vi "Test_Class.vi"() -> ()   [LabVIEW 2023, in "Picture2D.lvlib"]
uses:
  Picture2D/Picture2D.lvlib
  Circle/Circle.lvclass
  C:/GitHub/Picture2D/src/Shape/Shape.lvclass
  C:/GitHub/Picture2D/src/IDrawable/IDrawable.lvclass
  PointSpecialized/PointSpecialized.lvclass
  C:/GitHub/Picture2D/src/Point/Point.lvclass
  Collection/Collection.lvclass
  ColorHSL/ColorHSL.lvclass
  C:/GitHub/Picture2D/src/Color/Color.lvclass
  Pen/Pen.lvclass
  Picture/Image.lvclass
  Line/Line.lvclass
  Rectangle/Rectangle.lvclass
  C:/GitHub/Picture2D/src/Polygone/Polygone.lvclass
  Text/Text.lvclass
  C:/GitHub/Picture2D/src/Picture2D/Picture2D.lvclass
  Square/Square.lvclass
  RoundRectangle/RoundRectangle.lvclass
  C:/GitHub/Picture2D/src/Rectangle/Rectangle.lvclass
  Point/Point.lvclass
  Color/Color.lvclass
  Triangle/Triangle.lvclass
  Losange/Losange.lvclass
  TriangleR/TriangleR.lvclass
  C:/GitHub/Picture2D/src/Triangle/Triangle.lvclass
  Font/Font.lvclass
  UMLClass/UMLClass.lvclass
  TriangleL/TriangleL.lvclass
  TriangleB/TriangleB.lvclass
  GrayScaleImage/GrayScaleImage.lvclass
  C:/GitHub/Picture2D/src/Picture/Image.lvclass
  2DPictureControl/2DPictureControl.lvclass
  Font/Font.lvclass/Font.ctl
  UMLClass/UMLClass.lvclass/UMLClass.ctl
  PointSpecialized/PointSpecialized.lvclass/PointSpecialized.ctl
  Font/SetFontName.vi
  Font/SetSize.vi
  UMLClass/SetClassName.vi
  UMLClass/SetMethods.vi
  UMLClass/SetProperties.vi
  PointSpecialized/SetColor.vi
  PointSpecialized/SetPen.vi
panel:
  in  "Num Px":i16=1
  in  "Down":bool
  in  "Right":bool
  in  "Left":bool
  in  "Up":bool
  in  "Reinit":bool
  in  "Zoom Factor":dbl(slide)=1.0 scale=0.5..3.0
  in  "Fill":bool
  in  "Rotate (deg)":dbl(slide)=1.0 scale=-180.0..180.0
  in  "Point:y":i16(slide) scale=-100.0..100.0
  in  "Point:x":i16(slide) scale=-100.0..100.0
  in  "Scale Factor":dbl(slide)=1.0 scale=0.5..2.0
  out "2D Picture out":picture
  # "Move Absolute"
  # "Move Relative (1 px)"
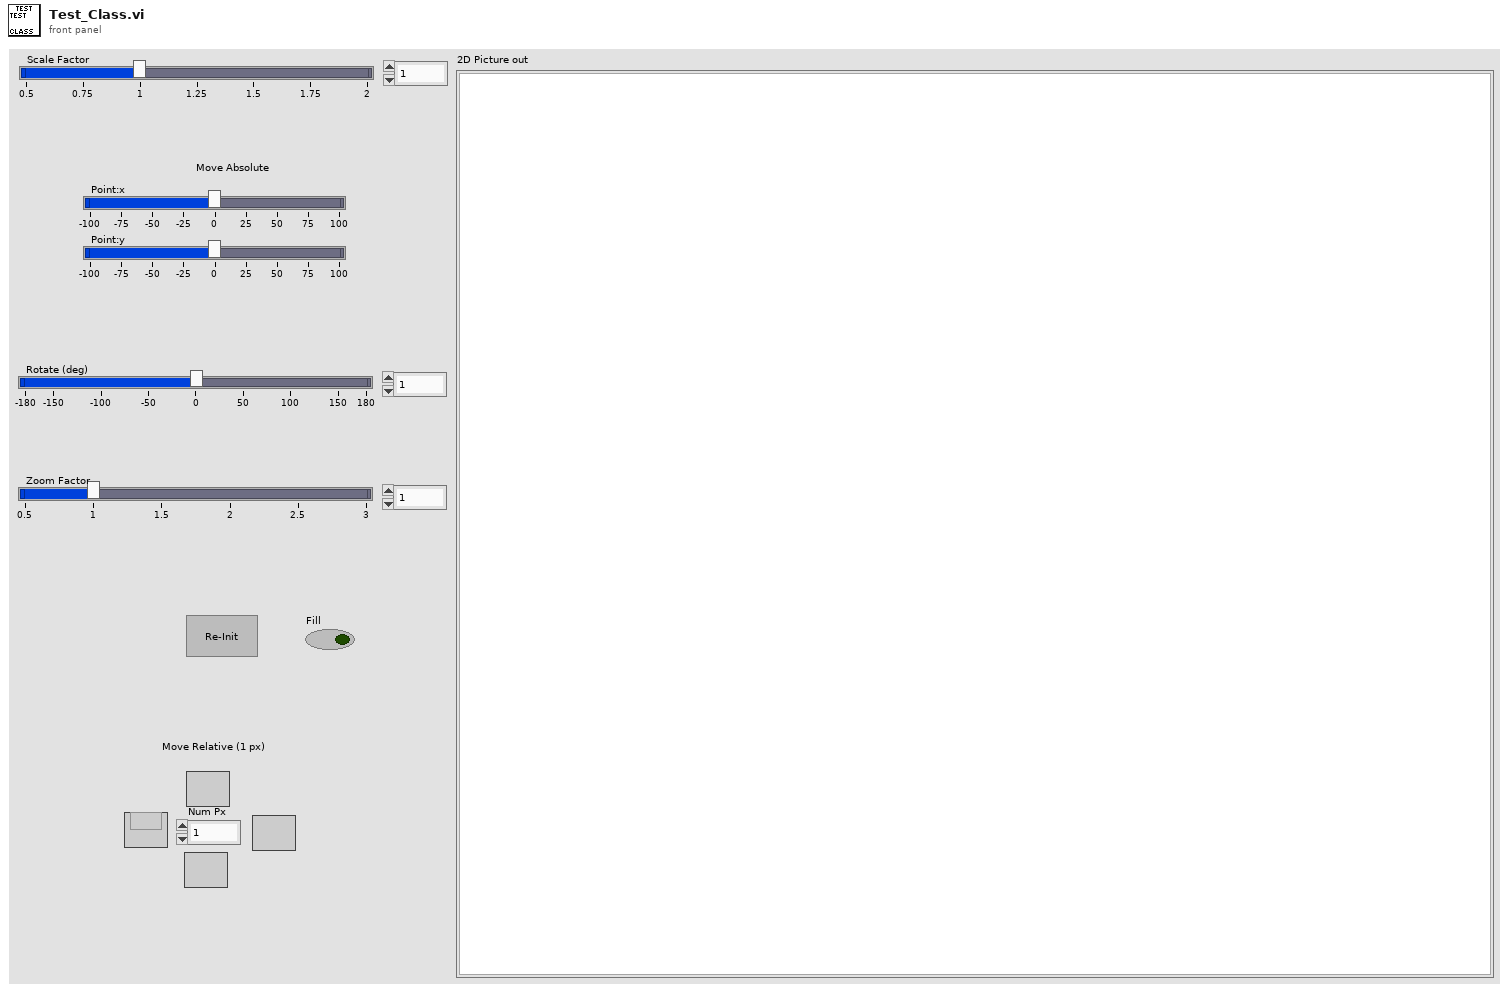
[diagram p1: front panel]
types:
  T1 = enum16{"User-specified Font", "Application Font", "System Font", "Dialog Font"}
  T2 = enum32{"Solid", "Dash", "Dot", "DashDot", "DashDotDot"}
  T3 = typedef "imagedata.ctl" = cluster{"image type":i32, "image depth":i32, "image":u8[], "mask":u8[], "colors":u32[], "Rectangle":cluster{"left":i16, "top":i16, "right":i16, "bottom":i16}}
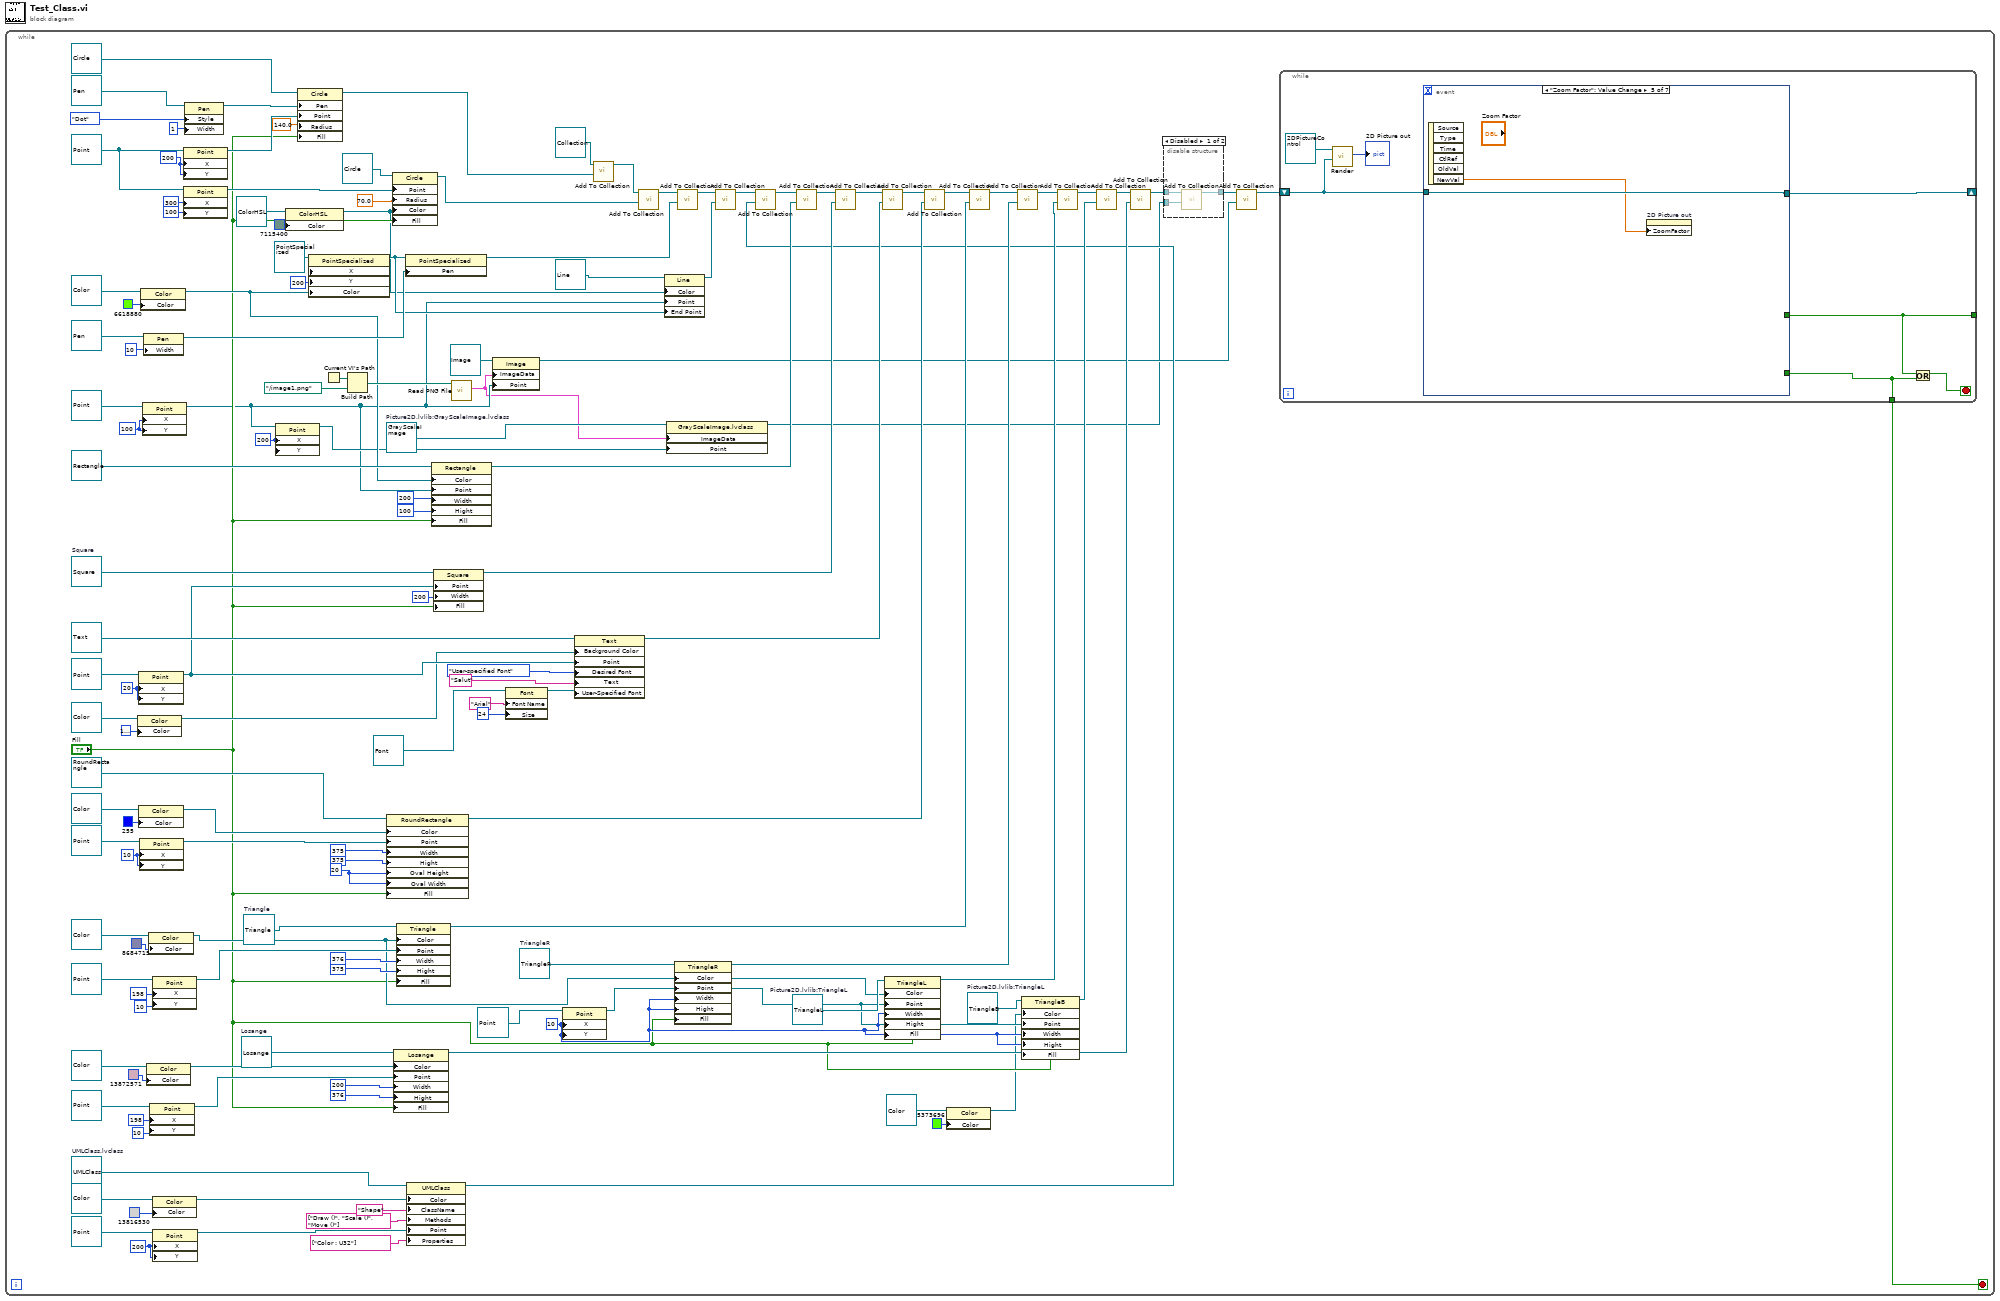
[diagram p0: block diagram]
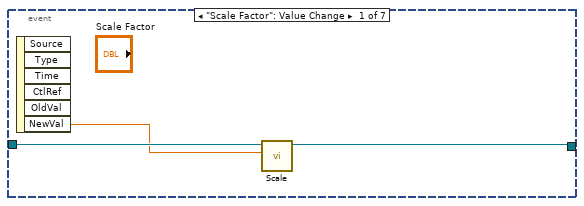
[diagram p3: hidden frame]
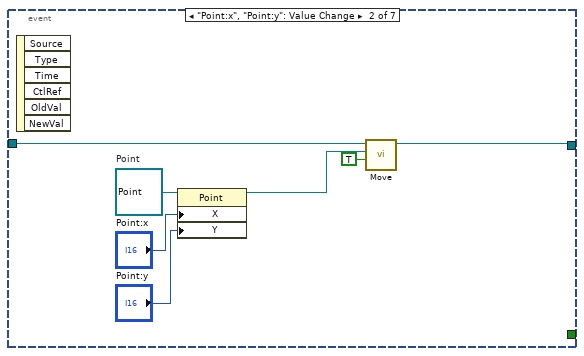
[diagram p4: hidden frame]
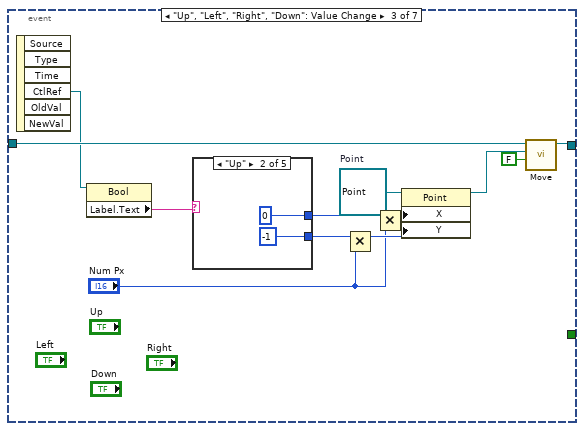
[diagram p5: hidden frame]
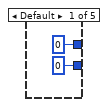
[diagram p6: hidden frame]
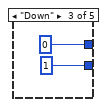
[diagram p7: hidden frame]
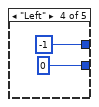
[diagram p8: hidden frame]
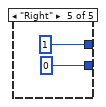
[diagram p9: hidden frame]
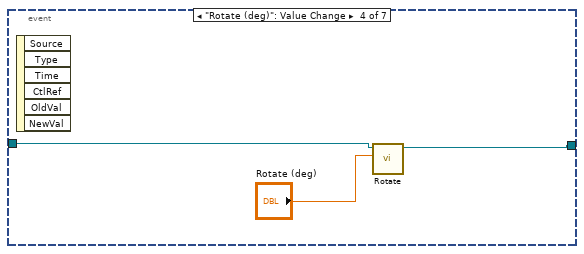
[diagram p10: hidden frame]
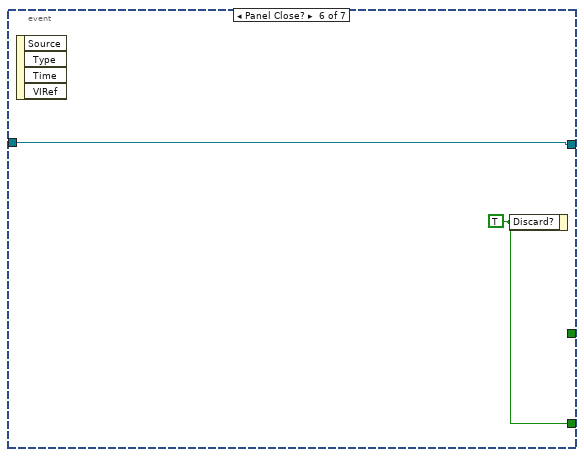
[diagram p11: hidden frame]
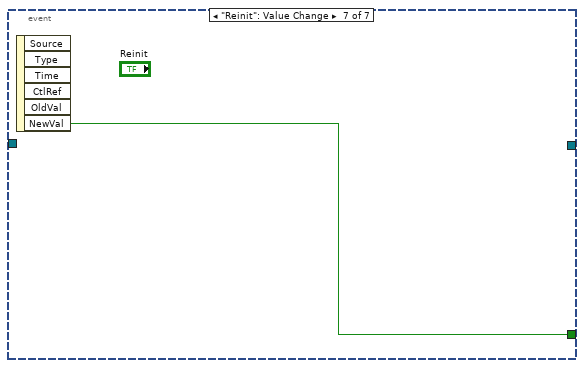
[diagram p12: hidden frame]
diagram:
  n1 = while {
    stop <- w1 stop-if-true
    w7 = i16 200 ("Point:X")
    w10 = refnum<class "GrayScaleImage.lvclass"> refnum  # Picture2D.lvlib:GrayScaleImage.lvclass
    w23 = refnum<class "TriangleB.lvclass"> refnum  # Picture2D.lvlib:TriangleL
    w26 = refnum<class "TriangleL.lvclass"> refnum  # Picture2D.lvlib:TriangleL
    w59 = refnum<class "UMLClass.lvclass"> refnum  # UMLClass.lvclass
    w20 = i16 10 ("Point:x")
    w35 = refnum<class "TriangleR.lvclass"> refnum  # TriangleR
    w44 = refnum<class "Losange.lvclass"> refnum  # Losange
    w68 = refnum<class "Triangle.lvclass"> refnum  # Triangle
    w72 = i16 200 ("x")
    w81 = i16 10 ("x")
    w82 = i16 20 ("Oval Height")
    w91 = refnum<class "Square.lvclass"> refnum  # Square
    w95 = i16 20 ("x")
    w113 = i16 100 ("x")
    w133 = i16 200 ("x")
    w140 = i16 200 ("x")
    w28 = refnum<class "Point.lvclass"> refnum ("Point")
    n2 = property class="Color"(reference=refnum<class "Color.lvclass"> refnum ("Color"), "Color"=u32 16777216) -> (reference out=w85:refnum<class "Color.lvclass">)  [unwired: 1 in, 1 out]
    n3 = property class="Point"(reference=refnum<class "Point.lvclass"> refnum ("Point"), "X"=w95, "Y"=w95) -> (reference out=w90:refnum<class "Point.lvclass">)  [unwired: 1 in, 1 out]
    n4 = property class="Color"(reference=refnum<class "Color.lvclass"> refnum ("Color"), "Color"=u32 255) -> (reference out=w76:refnum<class "Color.lvclass">)  [unwired: 1 in, 1 out]
    n5 = property class="Point"(reference=refnum<class "Point.lvclass"> refnum ("Point"), "X"=w81, "Y"=w81) -> (reference out=w79:refnum<class "Point.lvclass">)  [unwired: 1 in, 1 out]
    n6 = property class="Color"(reference=refnum<class "Color.lvclass"> refnum ("Color"), "Color"=u32 6618880) -> (reference out=w97:refnum<class "Color.lvclass">)  [unwired: 1 in, 1 out]
    n7 = property class="Point"(reference=refnum<class "Point.lvclass"> refnum ("Point"), "X"=w113, "Y"=w113) -> (reference out=w8:refnum<class "Point.lvclass">)  [unwired: 1 in, 1 out]
    n8 = property class="Pen"(reference=refnum<class "Pen.lvclass"> refnum ("Pen"), "Width"=u16 10) -> (reference out=w121:refnum<class "Pen.lvclass">)  [unwired: 1 in, 1 out]
    n9 = property class="Color"(reference=refnum<class "Color.lvclass"> refnum ("Color"), "Color"=u32 13872571) -> (reference out=w47:refnum<class "Color.lvclass">)  [unwired: 1 in, 1 out]
    n10 = property class="Color"(reference=refnum<class "Color.lvclass"> refnum ("Color"), "Color"=u32 8684715) -> (reference out=w22:refnum<class "Color.lvclass">)  [unwired: 1 in, 1 out]
    n11 = property class="Point"(reference=refnum<class "Point.lvclass"> refnum ("Point"), "X"=i16 198 ("x"), "Y"=i16 10 ("Point:y")) -> (reference out=w50:refnum<class "Point.lvclass">)  [unwired: 1 in, 1 out]
    n12 = property class="Point"(reference=refnum<class "Point.lvclass"> refnum ("Point"), "X"=i16 198 ("x"), "Y"=i16 10 ("Point:y")) -> (reference out=w63:refnum<class "Point.lvclass">)  [unwired: 1 in, 1 out]
    n13 = property class="Color"(reference=refnum<class "Color.lvclass"> refnum ("Color"), "Color"=u32 13816530) -> (reference out=w52:refnum<class "Color.lvclass">)  [unwired: 1 in, 1 out]
    n14 = property class="Point"(reference=refnum<class "Point.lvclass"> refnum ("Point"), "X"=w72, "Y"=w72) -> (reference out=w55:refnum<class "Point.lvclass">)  [unwired: 1 in, 1 out]
    n15 = property class="Point"(reference=w28, "X"=w140, "Y"=w140) -> (reference out=w138:refnum<class "Point.lvclass">)  [unwired: 1 in, 1 out]
    n16 = property class="Point"(reference=w28, "X"=i16 300 ("Point:x"), "Y"=i16 100 ("Point:y")) -> (reference out=w38:refnum<class "Point.lvclass">)  [unwired: 1 in, 1 out]
    n17 = property class="Pen"(reference=refnum<class "Pen.lvclass"> refnum ("Pen"), "Style"=T2."Dot", "Width"=u16 1) -> (reference out=w118:refnum<class "Pen.lvclass">)  [unwired: 1 in, 1 out]
    n18 = property class="Point"(reference=w8, "X"=w7, "Y"=w7) -> (reference out=w9:refnum<class "Point.lvclass">)  [unwired: 1 in, 1 out]
    n19 = property class="ColorHSL"(reference=refnum<class "ColorHSL.lvclass"> refnum ("Color"), "Color"=u32 7115400) -> (reference out=w11:refnum<class "ColorHSL.lvclass">)  [unwired: 1 in, 1 out]
    n20 = property class="Circle"(reference=refnum<class "Circle.lvclass"> refnum ("Circle.lvclass"), "Pen"=w118, "Point"=w138, "Radius"=140.0, "Fill"="Fill") -> (reference out=w136:refnum<class "Circle.lvclass">)  [unwired: 1 in, 1 out]
    n21 = property class="PointSpecialized"(reference=refnum<class "PointSpecialized.lvclass"> refnum ("Point"), "X"=w133, "Y"=w133, "Color"=w97) -> (reference out=w39:refnum<class "PointSpecialized.lvclass">)  [unwired: 1 in, 1 out]
    n22 = Current VI's Path() -> (path=w112:path)
    n23 = Build Path(base path=w112, name or relative path=path "../image1.png" ("path to PNG file")) -> (appended path=w110:path)
    n24 = property class="RoundRectangle"(reference=refnum<class "RoundRectangle.lvclass"> refnum ("RoundRectangle"), "Color"=w76, "Point"=w79, "Width"=i16 375, "Hight"=i16 375 ("Width"), "Oval Height"=w82, "Oval Width"=w82, "Fill"="Fill") -> (reference out=w73:refnum<class "RoundRectangle.lvclass">)  [unwired: 1 in, 1 out]
    n25 = property class="Circle"(reference=refnum<class "Circle.lvclass"> refnum ("Circle.lvclass"), "Point"=w38, "Radius"=70.0, "Color"=w11, "Fill"="Fill") -> (reference out=w131:refnum<class "Circle.lvclass">)  [unwired: 1 in, 1 out]
    n26 = property class="Losange"(reference=w44, "Color"=w47, "Point"=w50, "Width"=i16 200, "Hight"=i16 376 ("Width"), "Fill"="Fill") -> (reference out=w40:refnum<class "Losange.lvclass">)  [unwired: 1 in, 1 out]
    n27 = property class="Triangle"(reference=w68, "Color"=w22, "Point"=w63, "Width"=i16 376, "Hight"=i16 375 ("Width"), "Fill"="Fill") -> (reference out=w61:refnum<class "Triangle.lvclass">)  [unwired: 1 in, 1 out]
    n28 = property class="PointSpecialized"(reference=w39, "Pen"=w121) -> (reference out=w125:refnum<class "PointSpecialized.lvclass">)  [unwired: 1 in, 1 out]
    n29 = property class="UMLClass"(reference=w59, "Color"=w52, "ClassName"="Shape" ("Class Name"), "Methods"=string[] ["Draw ()", "Scale ()", "Move ()"], "Point"=w55, "Properties"=string[] ["Color : U32"]) -> (reference out=w12:refnum<class "UMLClass.lvclass">)  [unwired: 1 in, 1 out]
    n30 = property class="Rectangle"(reference=refnum<class "Rectangle.lvclass"> refnum ("Rectangle.lvclass"), "Color"=w97, "Point"=w8, "Width"=i16 200, "Hight"=i16 100, "Fill"="Fill") -> (reference out=w101:refnum<class "Rectangle.lvclass">)  [unwired: 1 in, 1 out]
    n31 = property class="Square"(reference=w91, "Point"=w90, "Width"=i16 200, "Fill"="Fill") -> (reference out=w88:refnum<class "Square.lvclass">)  [unwired: 1 in, 1 out]
    n32 = call <vilib>:"Read PNG File.vi"("path to PNG file"=w110) -> ("image data"=w4:T3)  [unwired: 8 in, 2 out]
    n33 = property class="Image"(reference=refnum<class "Image.lvclass"> refnum ("Image"), "ImageData"=w4, "Point"=w8) -> (reference out=w3:refnum<class "Image.lvclass">)  [unwired: 1 in, 1 out]
    n34 = property class="Font"(reference=refnum<class "Font.lvclass"> refnum ("User-Specified Font"), "Font Name"="Arial", "Size"=i16 24) -> (reference out=w31:refnum<class "Font.lvclass">)  [unwired: 1 in, 1 out]
    n35 = property class="Point"(reference=refnum<class "Point.lvclass"> refnum ("Point"), "X"=w20, "Y"=w20) -> (reference out=w21:refnum<class "Point.lvclass">)  [unwired: 1 in, 1 out]
    n36 = property class="Text"(reference=refnum<class "Text.lvclass"> refnum ("Text"), "Background Color"=w85, "Point"=w90, "Desired Font"=T1."User-specified Font", "Text"="Salut", "User-Specified Font"=w31) -> (reference out=w92:refnum<class "Text.lvclass">)  [unwired: 1 in, 1 out]
    n37 = call-dynamic "Add To Collection.vi"("IDrawable"=w136, "Collection in"=refnum<class "Collection.lvclass"> refnum) -> ("Collection out"=w130:refnum<class "Collection.lvclass">)  [unwired: 8 in, 1 out]
    n38 = call-dynamic "Add To Collection.vi"("IDrawable"=w131, "Collection in"=w130) -> ("Collection out"=w128:refnum<class "Collection.lvclass">)  [unwired: 8 in, 1 out]
    n39 = property class="Line"(reference=refnum<class "Line.lvclass"> refnum ("Line"), "Color"=w11, "Point"=w8, "End Point"=w39) -> (reference out=w106:refnum<class "Line.lvclass">)  [unwired: 1 in, 1 out]
    n40 = property class="GrayScaleImage.lvclass"(reference=w10, "ImageData"=w4, "Point"=w9) -> (reference out=w2:refnum<class "GrayScaleImage.lvclass">)  [unwired: 1 in, 1 out]
    n41 = property class="TriangleR"(reference=w35, "Color"=w22, "Point"=w21, "Width"=w20, "Hight"=w20, "Fill"="Fill") -> (reference out=w33:refnum<class "TriangleR.lvclass">)  [unwired: 1 in, 1 out]
    n42 = call-dynamic "Add To Collection.vi"("IDrawable"=w125, "Collection in"=w128) -> ("Collection out"=w108:refnum<class "Collection.lvclass">)  [unwired: 8 in, 1 out]
    n43 = call-dynamic "Add To Collection.vi"("IDrawable"=w106, "Collection in"=w108) -> ("Collection out"=w107:refnum<class "Collection.lvclass">)  [unwired: 8 in, 1 out]
    n44 = call-dynamic "Add To Collection.vi"("IDrawable"=w12, "Collection in"=w107) -> ("Collection out"=w102:refnum<class "Collection.lvclass">)  [unwired: 8 in, 1 out]
    n45 = call-dynamic "Add To Collection.vi"("IDrawable"=w101, "Collection in"=w102) -> ("Collection out"=w100:refnum<class "Collection.lvclass">)  [unwired: 8 in, 1 out]
    n46 = call-dynamic "Add To Collection.vi"("IDrawable"=w88, "Collection in"=w100) -> ("Collection out"=w99:refnum<class "Collection.lvclass">)  [unwired: 8 in, 1 out]
    n47 = call-dynamic "Add To Collection.vi"("IDrawable"=w92, "Collection in"=w99) -> ("Collection out"=w84:refnum<class "Collection.lvclass">)  [unwired: 8 in, 1 out]
    n48 = property class="TriangleL"(reference=w26, "Color"=w22, "Point"=w21, "Width"=w20, "Hight"=w20, "Fill"="Fill") -> (reference out=w24:refnum<class "TriangleL.lvclass">)  [unwired: 1 in, 1 out]
    n49 = call-dynamic "Add To Collection.vi"("IDrawable"=w73, "Collection in"=w84) -> ("Collection out"=w62:refnum<class "Collection.lvclass">)  [unwired: 8 in, 1 out]
    n50 = property class="Color"(reference=refnum<class "Color.lvclass"> refnum ("Color"), "Color"=u32 5373696) -> (reference out=w14:refnum<class "Color.lvclass">)  [unwired: 1 in, 1 out]
    n51 = call-dynamic "Add To Collection.vi"("IDrawable"=w61, "Collection in"=w62) -> ("Collection out"=w34:refnum<class "Collection.lvclass">)  [unwired: 8 in, 1 out]
    n52 = call-dynamic "Add To Collection.vi"("IDrawable"=w33, "Collection in"=w34) -> ("Collection out"=w25:refnum<class "Collection.lvclass">)  [unwired: 8 in, 1 out]
    n53 = property class="TriangleB"(reference=w23, "Color"=w14, "Point"=w21, "Width"=w20, "Hight"=w20, "Fill"="Fill") -> (reference out=w16:refnum<class "TriangleB.lvclass">)  [unwired: 1 in, 1 out]
    n54 = call-dynamic "Add To Collection.vi"("IDrawable"=w24, "Collection in"=w25) -> ("Collection out"=w18:refnum<class "Collection.lvclass">)  [unwired: 8 in, 1 out]
    n55 = call-dynamic "Add To Collection.vi"("IDrawable"=w16, "Collection in"=w18) -> ("Collection out"=w17:refnum<class "Collection.lvclass">)  [unwired: 8 in, 1 out]
    n56 = call-dynamic "Add To Collection.vi"("IDrawable"=w40, "Collection in"=w17) -> ("Collection out"=w41:refnum<class "Collection.lvclass">)  [unwired: 8 in, 1 out]
    n57 = disable-structure shown="Disabled" {
      disable-tunnel: w41 -> [w143 w144]
      disable-tunnel: [w142 w144] -> w6
      disable-tunnel: w2 -> [w141 _]
      frame Disabled {
        n58 = call-dynamic "Add To Collection.vi"("IDrawable"=w141, "Collection in"=w143) -> ("Collection out"=w142:refnum<class "Collection.lvclass">)  [unwired: 8 in, 1 out]
      }
      frame Enabled {
        # "Grayscale\nSlow to Render"
      }
    }
    n59 = call-dynamic "Add To Collection.vi"("IDrawable"=w3, "Collection in"=w6) -> ("Collection out"=w5:refnum<class "Collection.lvclass">)  [unwired: 8 in, 1 out]
    n60 = while {
      shift-right: [w149] -> _
      shift-left: w5 -> [w148]
      tunnel: [w146] -> _
      tunnel: [w145] -> w1
      stop <- w147 stop-if-true
      n61 = call-dynamic "Render.vi"("IDrawable"=w148, "2DPictureControl in"=refnum<class "2DPictureControl.lvclass"> refnum ("2DPictureControl.lvclass")) -> ("2D Picture out"=→"2D Picture out":picture)  [unwired: 7 in, 2 out]
      n62 = event shown="[4] \"Zoom Factor\": Value Change" {
        selector: _ -> [_ _ _ _ _ _ _]
        dyn-events: _ -> [_ _ _ _ _ _ _]
        timeout: _ -> [_ _ _ _ _ _ _]
        tunnel: w148 -> [w154 w157 w171 w185 w188 w189 _]
        tunnel: [w153 w156 w170 w186 w188 w189 _] -> w149
        tunnel: [_ _ _ _ _ w190 _] -> w145
        tunnel: [_ _ _ _ _ _ w191] -> w146
        event "Scale Factor": Value Change {
          n63 = event-data() -> ("NewVal"=w152:dbl)  [unwired: 1 in, 5 out]
          n64 = call-dynamic "Scale.vi"("Scale Factor"=w152, "Collection in"=w154) -> ("Collection out"=w153:refnum<class "Collection.lvclass">)  [unwired: 8 in, 1 out]
        }
        event "Point:x", "Point:y": Value Change {
          w158 = refnum<class "Point.lvclass"> refnum  # Point
          n65 = event-data() -> ()  [unwired: 1 in, 6 out]
          n66 = property class="Point"(reference=w158, "X"="Point:x", "Y"="Point:y") -> (reference out=w159:refnum<class "Point.lvclass">)  [unwired: 1 in, 1 out]
          n67 = call-dynamic "Move.vi"("Absolute (T)"=TRUE, "Point"=w159, "Collection in"=w157) -> ("Collection out"=w156:refnum<class "Collection.lvclass">)  [unwired: 7 in, 1 out]
        }
        event "Up", "Left", "Right", "Down": Value Change {
          w172 = refnum<class "Point.lvclass"> refnum  # Point
          n68 = event-data() -> ("CtlRef"=w168:refnum<vi>)  [unwired: 1 in, 5 out]
          n69 = property class="Bool"(reference=w168) -> ("Label.Text"=w167:string)  [unwired: 1 in, 2 out]
          n70 = case shown="\"Up\"" w167 {
            tunnel: [i16 0 i16 0 i16 0 i16 -1 i16 1] -> w166
            tunnel: [i16 0 i16 -1 i16 1 i16 0 i16 0] -> w165
            frame Default {
            }
            frame "Up" {
            }
            frame "Down" {
            }
            frame "Left" {
            }
            frame "Right" {
            }
          }
          n71 = Multiply(x=w165, y="Num Px") -> (x*y=w164:i16)
          n72 = Multiply(x=w166, y="Num Px") -> (x*y=w163:i16)
          n73 = property class="Point"(reference=w172, "X"=w163, "Y"=w164) -> (reference out=w173:refnum<class "Point.lvclass">)  [unwired: 1 in, 1 out]
          n74 = call-dynamic "Move.vi"("Absolute (T)"=FALSE, "Point"=w173, "Collection in"=w171) -> ("Collection out"=w170:refnum<class "Collection.lvclass">)  [unwired: 7 in, 1 out]
        }
        event "Rotate (deg)": Value Change {
          n75 = event-data() -> ()  [unwired: 1 in, 6 out]
          n76 = call-dynamic "Rotate.vi"("Angle (deg)"="Rotate (deg)", "Collection in"=w185) -> ("Collection out"=w186:refnum<class "Collection.lvclass">)  [unwired: 8 in, 1 out]
        }
        event "Zoom Factor": Value Change {
          n77 = event-data() -> ("NewVal"=w187:dbl)  [unwired: 1 in, 5 out]
          n78 = property on="2D Picture out" class="Pict"("ZoomFactor"=w187) -> ()  [unwired: 2 in, 2 out]
        }
        event Panel Close? {
          w190 = TRUE ("Discard?")
          n79 = event-data() -> ()  [unwired: 1 in, 4 out]
          n80 = event-data("Discard?"=w190) -> ()  [unwired: 1 in, 1 out]
        }
        event "Reinit": Value Change {
          n81 = event-data() -> ("NewVal"=w191:bool)  [unwired: 1 in, 5 out]
        }
      }
      n82 = Or(x=w146, y=w145) -> (x .or. y?=w147:bool)
    }
  }
